vi "Transform_Inverse.vi"(11 "inTRANSFORM":T1={"TRANSLATION"={"X"=0.0, "Y"=0.0}, "ROTATION"={"VALUE"=0.0, "COS"=1.0, "SIN"=0.0}}) -> (3 "TRANSFORM":T1)   [LabVIEW 2019, in "Trajectory_Library.lvlib"]
doc: "Invert the transformation. This is useful for undoing a transformation.\n\nParameters:\n - IN TRANSFORM - This TRANSFORM data structure\n\nResults:\n - OUT TRANSFORM - The inverted transformation."
uses:
  Trajectory_Library.lvlib
  TRANSFORM2D.ctl
  TRANSLATION2D.ctl
  ROTATION2D.ctl
  Translation_Create.vi
  Rotation_CreateAngle.vi
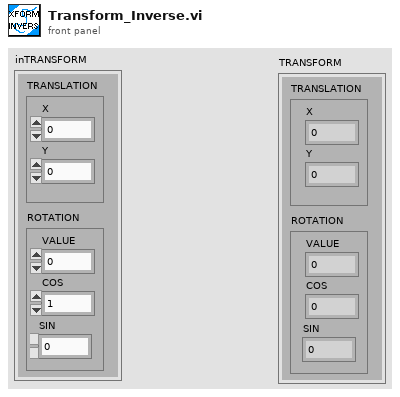
[diagram p1: front panel]
types:
  T1 = typedef "Trajectory_Library.lvlib/TRANSFORM2D.ctl" = cluster{"TRANSLATION":T2, "ROTATION":T3}
  T2 = typedef "Trajectory_Library.lvlib/TRANSLATION2D.ctl" = cluster{"X":dbl, "Y":dbl}
  T3 = typedef "Trajectory_Library.lvlib/ROTATION2D.ctl" = cluster{"VALUE":dbl, "COS":dbl, "SIN":dbl}
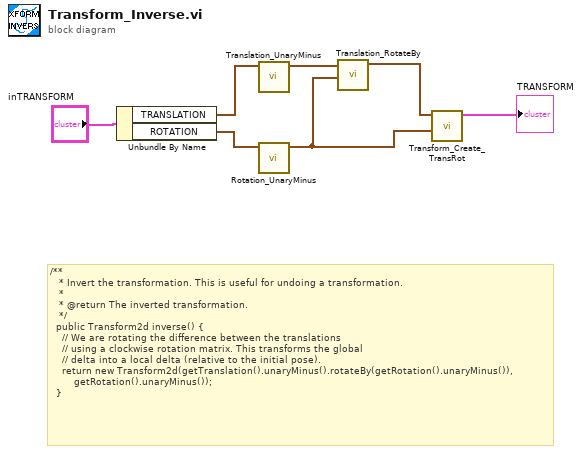
[diagram p0: block diagram]
diagram:
  # "/**\n   * Invert the transformation. This is useful for undoing a transformation.\n   *\n   * @return The inverted transformation.\n   */\n  public Transform2d inverse() {\n    // We are rotating the difference between the translations\n    // using a clockwise rotation matrix. This transforms the global\n    // delta into a local delta (relative to the initial pose).\n    return new Transform2d(getTranslation().unaryMinus().rotateBy(getRotation().unaryMinus()),\n        getRotation().unaryMinus());\n  }"
  n1 = Unbundle By Name("inTRANSFORM") -> ("TRANSLATION"=w5:T2, "ROTATION"=w4:T3)
  n2 = call "Translation_UnaryMinus.vi"("In Translation"=w5) -> ("Out Translation"=w3:T2)  [unwired: 10 in]
  n3 = call "Rotation_UnaryMinus.vi"("in ROTATION"=w4) -> ("out ROTATION"=w1:T3)  [unwired: 10 in]
  n4 = call "Translation_RotateBy.vi"("other Rotation"=w1, "In Translation"=w3) -> ("Out Translation"=w2:T2)  [unwired: 9 in]
  n5 = call "Transform_Create_TransRot.vi"("ROTATION"=w1, "TRANSLATION"=w2) -> ("TRANSFORM"=→"TRANSFORM":T1)  [unwired: 9 in]
